vi "SET_ActiveTool.vi"(8 "error in (no error)":errorcluster, 10 "Radio Buttons":T1, 11 "Tools Paint.lvclass in":refnum<class "Tools Paint.lvclass">) -> (0 "error out":errorcluster, 3 "Tools Paint.lvclass out":refnum<class "Tools Paint.lvclass">)   [LabVIEW 2020, in "Tools Paint.lvclass"]
uses:
  Tools Paint.lvclass
  Tools Paint.lvclass/Tools Paint.ctl
  Controls/Circle.ctl
  Controls/Dropper.ctl
  Controls/FCircle.ctl
  Controls/Fill.ctl
  Controls/FRect.ctl
  Controls/Line.ctl
  Controls/Move.ctl
  Controls/Pen.ctl
  Controls/IERect.ctl
  Controls/Rubber.ctl
  Controls/Selection.ctl
  Controls/Text.ctl
  Controls/Tools.ctl
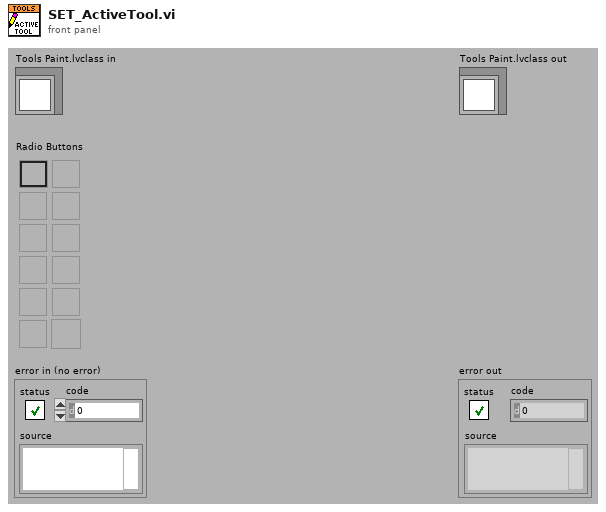
[diagram p1: front panel]
types:
  T1 = typedef "Tools.ctl" = enum32{"Pencil", "Line", "Dropper", "Fill", "Rectangle", "Filled Rectangle", "Ellipse", "Filled Ellipse", "Eraser", "Text", "Select", "Move"}
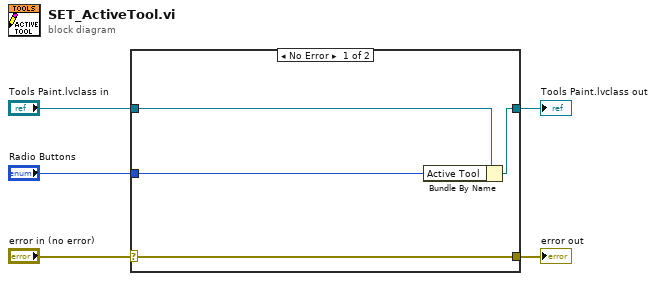
[diagram p0: block diagram]
diagram:
  n1 = case shown="No Error" "error in (no error)" {
    selector: "error in (no error)" -> [w9 w10]
    tunnel: [w9 w10] -> w4
    tunnel: [w7 w11] -> w2
    tunnel: "Tools Paint.lvclass in" -> [w8 w11]
    tunnel: "Radio Buttons" -> [w6 _]
    frame No Error {
      n2 = Bundle By Name(cluster=w8, "Active Tool"=w6) -> (w7:refnum<class "Tools Paint.lvclass">)
    }
    frame Error {
    }
  }
  "error out" <- w4
  "Tools Paint.lvclass out" <- w2
